vi "TPG361_Main.vi"() -> ()   [LabVIEW 2019]
uses:
  TPG361_Global.vi
panel:
  out "Chart":waveform(dbl)[](graph)
  out "status_log":bool caption="Status"
  out "status_read":bool caption="Status"
  in  "Logging":bool=TRUE
  out "PKR 361":dbl format="%_3e"
  in  "stop":bool
  out "Last Measurement":timestamp format="%<%Y-%m-%d %H:%M:%S>T"
  in  "VISA":refnum<visa-resource-name>="COM32"
  in  "Measurement Rate (ms)":i32=5000
  # "TPG361"
  # "IVC Pressure"
  # "Torr"
  # "Chart-Axis Control"
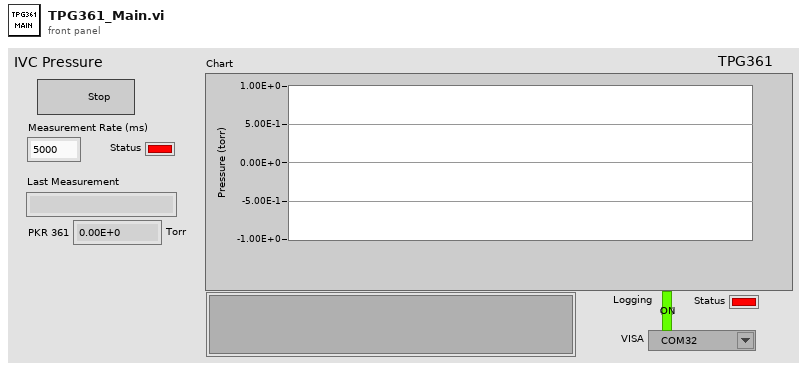
[diagram p1: front panel]
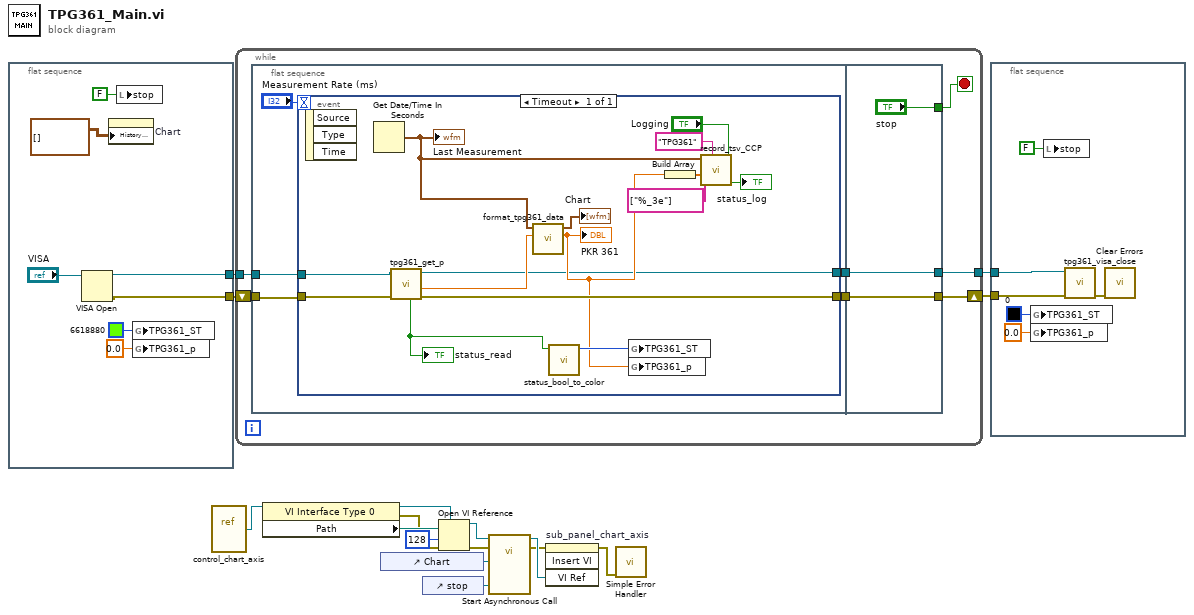
[diagram p0: block diagram]
diagram:
  n1 = flat-sequence {
    tunnel: [w21] -> w16
    tunnel: [w20] -> w15
    frame #0 {
      n2 = VISA Open(VISA resource name="VISA") -> (VISA resource name=w21:refnum<visa-resource-name>, error out=w20:errorcluster)  [unwired: 4 in]
      n3 = property on="Chart" class="WFChart (strict)"("History Data"=waveform(dbl)[][] []) -> ()  [unwired: 2 in, 2 out]
      n4 = local write "stop"(FALSE ("stop")) -> ()
      n5 = global write "TPG361_Global.vi" "TPG361_ST"(u32 6618880 ("TPG361_ST")) -> ()
      n6 = global write "TPG361_Global.vi" "TPG361_p"(0.0 ("TPG361_p")) -> ()
    }
  }
  n7 = vi-ref "control_chart_axis.vi"() -> (w13:refnum<vi>)
  n8 = while {
    tunnel: w16 -> [w30]
    tunnel: [w29] -> w2
    shift-right: [w25] -> w1
    shift-left: w15 -> [w28]
    stop <- w26 stop-if-true
    n9 = flat-sequence {
      tunnel: w30 -> [w34]
      tunnel: w28 -> [w32]
      tunnel: [w33] -> w27
      tunnel: [w31] -> w24
      tunnel: [w53] -> w29
      tunnel: w27 -> [w53]
      tunnel: ["stop"] -> w26
      tunnel: [w52] -> w25
      tunnel: w24 -> [w52]
      frame #0 {
        n10 = event shown="[0] Timeout" {
          selector: _ -> [_]
          dyn-events: _ -> [_]
          timeout: "Measurement Rate (ms)" -> [_]
          tunnel: w34 -> [w44]
          tunnel: [w36] -> w33
          tunnel: w32 -> [w47]
          tunnel: [w42] -> w31
          event Timeout {
            n11 = event-data() -> ()  [unwired: 1 in, 3 out]
            n12 = Get Date/Time In Seconds() -> (seconds since 1Jan1904=w45:timestamp)
            "Last Measurement" <- w45
            n13 = call "tpg361_get_p.vi"("err_in"=w47, "visa_in"=w44) -> ("err_out"=w42:errorcluster, "pressure"=w43:dbl, "visa_out"=w36:refnum<visa-resource-name>, "status_all"=w38:bool)  [unwired: 5 in, 1 out]
            "status_read" <- w38
            n14 = call "format_tpg361_data.vi"("pressure"=w43, "time"=w45) -> ("pressure_out"=w37:dbl, "waveform_array"=→"Chart":waveform(dbl)[])  [unwired: 8 in]
            "PKR 361" <- w37
            n15 = call "status_bool_to_color.vi"("status_bool_1"=w38) -> ("status_color"=w39:u32)  [unwired: 10 in]
            n16 = global write "TPG361_Global.vi" "TPG361_ST"(w39) -> ()
            n17 = global write "TPG361_Global.vi" "TPG361_p"(w37) -> ()
            n18 = Build Array(w37) -> (w41:dbl[])
            n19 = call "record_tsv_CCP.vi"("logging_on"="Logging", "folder_name"="TPG361", "format_array"=string[] ["%_3e"], "value_array"=w41, "time"=w45) -> ("status_log"=→"status_log":bool)  [unwired: 5 in, 1 out]
          }
        }
      }
      frame #1 {
      }
    }
  }
  n20 = property class="VI Interface Type 0"(reference=w13) -> (reference out=w11:refnum<vi>, error out=w10:errorcluster, "Path"=w14:path)  [unwired: 1 in]
  n21 = control-ref of="Chart"() -> (w3:refnum<vi>)
  n22 = control-ref of="stop"() -> (w4:refnum<vi>)
  n23 = Open VI Reference(type specifier VI Refnum (for type only)=w11, vi path=w14, options=128, error in (no error)=w10) -> (vi reference=w5:refnum<vi>, error out=w6:errorcluster)  [unwired: 2 in]
  n24 = call-by-ref "Start Asynchronous Call"(reference=w5, error in=w6, "stop"=w4, "chart_1"=w3) -> (reference out=w9:refnum<vi>, error out=w8:errorcluster)  [unwired: 10 in]
  n25 = invoke on="sub_panel_chart_axis" class="SubPnl" method="Insert VI"(error in=w8, "VI Ref"=w9) -> (error out=w7:errorcluster)  [unwired: 2 in, 3 out]
  n26 = call <vilib>:"Simple Error Handler.vi"("error in (no error)"=w7) -> ()  [unwired: 4 in, 5 out]
  n27 = flat-sequence {
    tunnel: w2 -> [w59]
    tunnel: w1 -> [w58]
    frame #0 {
      n28 = global write "TPG361_Global.vi" "TPG361_ST"(u32 0 ("TPG361_ST")) -> ()
      n29 = global write "TPG361_Global.vi" "TPG361_p"(0.0 ("TPG361_p")) -> ()
      n30 = local write "stop"(FALSE ("stop")) -> ()
      n31 = call "tpg361_visa_close.vi"("error in (no error)"=w58, "VISA session"=w59) -> ("error out"=w54:errorcluster)  [unwired: 9 in]
      n32 = call <vilib>:"Clear Errors.vi"("error in (no error)"=w54) -> ()  [unwired: 5 in, 2 out]
    }
  }
